vi "script-Matlab-proj.vi"(0 "Xr":i32[](array[numeric])=[230, 230, 230, 230, 230, 230, 230, 230, 230, 230, 230, 230, 230, 230, 230, 230, 230, 230, 230, 230, 230, 230, 230, 230, 230, 230, 230, 230, 230, 230, 230, 230, 230, 230, 230, 230, 230, 230, 230, 230, 230, 230, 230, 230, 230, 230, 230, 230, 230, 230, 230, 230, 230, 230, 230, 230, 230, 230, 230, 230, 230, 230, 230, 230, 230, 230, 230, 230, 230, 230, 225, 221, 213, 210, 206, 203, 195, 192, 189, 185, 179, 175, 172, 168, 162, 158, 155, 151, 145, 142, 139, 136, 129, 128, 131, 131, 136, 137, 139, 140, 144, 145, 147, 149, 151, 153, 155, 156, 159, 161, 163, 164, 167, 168, 170, 172, 175, 176, 178, 179, 182, 183, 184, 186, 189, 190, 191, 193, 195, 196, 198, 199, 201, 202, 203, 205, 207, 209, 209, 211, 213, 213], 1 "Xw":i32[](array[numeric])=[239, 239, 239, 239, 245, 265, 284, 302, 340, 359, 378, 397, 434, 453, 472, 491, 527, 545, 563, 580, 616, 635, 652, 670, 705, 723, 720, 705, 676, 663, 651, 641, 621, 612, 603, 595, 578, 569, 560, 552, 535, 526, 518, 509, 492, 484, 476, 467, 451, 442, 434, 426, 409, 401, 393, 385, 368, 360, 352, 344, 328, 320, 312, 304, 288, 280, 272, 264, 248, 241, 237, 234, 227, 223, 219, 215, 208, 204, 200, 197, 189, 186, 182, 178, 171, 167, 164, 160, 153, 149, 146, 143, 136, 132, 129, 128, 133, 135, 137, 138, 142, 144, 146, 147, 151, 152, 154, 156, 159, 161, 162, 164, 167, 168, 169, 171, 173, 175, 176, 178, 180, 181, 182, 184, 186, 187, 188, 190, 192, 193, 194, 195, 197, 198, 199, 200, 202, 203, 204, 205, 207, 208], 3 "filename":string="T5", 5 "Yr":i32[](array[numeric])=[319, 319, 319, 319, 319, 319, 319, 319, 319, 319, 319, 319, 319, 319, 319, 319, 319, 319, 319, 319, 319, 319, 319, 319, 319, 319, 319, 319, 319, 319, 319, 319, 319, 319, 319, 319, 319, 319, 319, 319, 319, 319, 319, 319, 319, 319, 319, 319, 319, 319, 319, 319, 319, 319, 319, 319, 319, 319, 319, 319, 319, 319, 319, 319, 319, 319, 319, 319, 319, 319, 315, 312, 306, 303, 301, 297, 291, 290, 287, 285, 280, 277, 274, 271, 267, 264, 261, 259, 255, 252, 249, 247, 242, 239, 239, 237, 233, 231, 229, 229, 225, 223, 222, 221, 217, 216, 214, 213, 210, 209, 207, 206, 203, 202, 200, 198, 195, 194, 193, 191, 189, 187, 187, 185, 183, 181, 180, 179, 176, 175, 174, 173, 171, 169, 168, 167, 165, 163, 163, 161, 159, 159], 9 "Xy":i32[](array[numeric])=[243, 243, 243, 243, 243, 243, 243, 243, 243, 243, 243, 243, 243, 243, 243, 243, 243, 243, 243, 243, 243, 243, 243, 243, 243, 243, 243, 243, 243, 243, 243, 243, 243, 243, 243, 243, 243, 243, 243, 243, 243, 243, 243, 243, 243, 243, 243, 243, 243, 243, 243, 243, 243, 243, 243, 243, 243, 243, 243, 243, 243, 243, 243, 243, 243, 243, 243, 243, 243, 243, 243, 243, 243, 243, 243, 243, 243, 243, 243, 243, 243, 243, 243, 243, 243, 243, 243, 243, 243, 243, 243, 243, 243, 243, 243, 243, 243, 243, 243, 243, 243, 243, 243, 243, 243, 243, 243, 243, 243, 243, 243, 243, 243, 243, 243, 243, 243, 243, 243, 243, 243, 243, 243, 243, 243, 243, 243, 243, 243, 243, 243, 243, 242, 242, 242, 242, 242, 242, 242, 242, 242, 242], 10 "error in":errorcluster, 11 "Yy":i32[](array[numeric])=[344, 344, 344, 344, 344, 344, 344, 344, 344, 344, 344, 344, 344, 344, 344, 344, 344, 344, 344, 344, 344, 344, 344, 344, 344, 344, 344, 344, 344, 344, 344, 344, 344, 344, 344, 344, 344, 344, 344, 344, 344, 344, 344, 344, 344, 344, 344, 344, 344, 344, 344, 344, 344, 344, 344, 344, 344, 344, 344, 344, 344, 344, 344, 344, 344, 344, 344, 344, 344, 344, 344, 344, 344, 344, 344, 344, 344, 344, 344, 344, 344, 344, 344, 344, 344, 344, 344, 344, 344, 344, 344, 344, 344, 344, 344, 344, 344, 344, 344, 344, 344, 344, 344, 344, 344, 344, 344, 344, 344, 344, 344, 344, 344, 344, 344, 344, 344, 344, 344, 344, 344, 344, 344, 344, 344, 344, 344, 344, 344, 344, 344, 344, 344, 344, 344, 344, 344, 344, 344, 344, 344, 344], 12 "Yw":i32[](array[numeric])=[368, 368, 368, 368, 369, 370, 372, 373, 377, 380, 382, 383, 387, 389, 391, 392, 391, 390, 389, 387, 386, 385, 384, 383, 381, 380, 382, 385, 390, 392, 391, 389, 386, 384, 383, 382, 379, 378, 376, 375, 373, 371, 370, 369, 367, 365, 364, 362, 360, 359, 357, 356, 354, 352, 351, 350, 347, 346, 345, 343, 341, 339, 338, 337, 335, 333, 332, 331, 328, 327, 329, 332, 336, 337, 339, 341, 344, 346, 348, 350, 353, 355, 356, 358, 361, 363, 365, 366, 369, 371, 373, 374, 378, 379, 381, 382, 383, 383, 384, 385, 386, 387, 388, 388, 390, 390, 391, 391, 392, 393, 393, 393, 393, 393, 393, 392, 391, 391, 391, 390, 390, 390, 389, 389, 388, 388, 388, 387, 387, 386, 386, 386, 386, 385, 385, 385, 384, 384, 384, 383, 383, 383], 13 "Line":string=".-", 14 "rgb1":string="68\t255\t18\n", 15 "rgb2":string="149\t0\t239\n") -> (4 "error out":errorcluster, 6 "matlab path":path=path "/Users/jammans/Documents/projet-prog/AnalyseT5.m")   [LabVIEW 2025]
panel:
  out "script matlab":string="% Auteurs: Rafaela Rebeiz, Jamil Mansour, Makram Fadel, Kevin Jandri\nclear\nclose all\nfilename = \"T5\";\nline = \".-\";\nrgb1 = [68\t255\t18\n];\nrgb2 = [149\t0\t239\n];\nXr=[230,230,230,230,230,230,230,230,230,230,230,230,230,230,230,230,230,230,230,230,230,230,230,230,230,230,230,230,230,230,230,230,230,230,230,230,230,230,230,230,230,230,230,230,230,230,230,230,230,230,230,230,230,230,230,230,230,230,230,230,230,230,230,230,230,230,230,230,230,230,225,221,213,210,206,203,195,192,189,185,179,175,172,168,162,158,155,151,145,142,139,136,129,128,131,131,136,137,139,140,144,145,147,149,151,153,155,156,159,161,163,164,167,168,170,172,175,176,178,179,182,183,184,186,189,190,191,193,195,196,198,199,201,202,203,205,207,209,209,211,213,213\n];\nYr=[319,319,319,319,319,319,319,319,319,319,319,319,319,319,319,319,319,319,319,319,319,319,319,319,319,319,319,319,319,319,319,319,319,319,319,319,319,319,319,319,319,319,319,319,319,319,319,319,319,319,319,319,319,319,319,319,319,319,319,319,319,319,319,319,319,319,319,319,319,319,315,312,306,303,301,297,291,290,287,285,280,277,274,271,267,264,261,259,255,252,249,247,242,239,239,237,233,231,229,229,225,223,222,221,217,216,214,213,210,209,207,206,203,202,200,198,195,194,193,191,189,187,187,185,183,181,180,179,176,175,174,173,171,169,168,167,165,163,163,161,159,159\n];\nXy=[243,243,243,243,243,243,243,243,243,243,243,243,243,243,243,243,243,243,243,243,243,243,243,243,243,243,243,243,243,243,243,243,243,243,243,243,243,243,243,243,243,243,243,243,243,243,243,243,243,243,243,243,243,243,243,243,243,243,243,243,243,243,243,243,243,243,243,243,243,243,243,243,243,243,243,243,243,243,243,243,243,243,243,243,243,243,243,243,243,243,243,243,243,243,243,243,243,243,243,243,243,243,243,243,243,243,243,243,243,243,243,243,243,243,243,243,243,243,243,243,243,243,243,243,243,243,243,243,243,243,243,243,242,242,242,242,242,242,242,242,242,242\n];\nYy=[344,344,344,344,344,344,344,344,344,344,344,344,344,344,344,344,344,344,344,344,344,344,344,344,344,344,344,344,344,344,344,344,344,344,344,344,344,344,344,344,344,344,344,344,344,344,344,344,344,344,344,344,344,344,344,344,344,344,344,344,344,344,344,344,344,344,344,344,344,344,344,344,344,344,344,344,344,344,344,344,344,344,344,344,344,344,344,344,344,344,344,344,344,344,344,344,344,344,344,344,344,344,344,344,344,344,344,344,344,344,344,344,344,344,344,344,344,344,344,344,344,344,344,344,344,344,344,344,344,344,344,344,344,344,344,344,344,344,344,344,344,344\n];\nXw=[239,239,239,239,245,265,284,302,340,359,378,397,434,453,472,491,527,545,563,580,616,635,652,670,705,723,720,705,676,663,651,641,621,612,603,595,578,569,560,552,535,526,518,509,492,484,476,467,451,442,434,426,409,401,393,385,368,360,352,344,328,320,312,304,288,280,272,264,248,241,237,234,227,223,219,215,208,204,200,197,189,186,182,178,171,167,164,160,153,149,146,143,136,132,129,128,133,135,137,138,142,144,146,147,151,152,154,156,159,161,162,164,167,168,169,171,173,175,176,178,180,181,182,184,186,187,188,190,192,193,194,195,197,198,199,200,202,203,204,205,207,208\n];\nYw=[368,368,368,368,369,370,372,373,377,380,382,383,387,389,391,392,391,390,389,387,386,385,384,383,381,380,382,385,390,392,391,389,386,384,383,382,379,378,376,375,373,371,370,369,367,365,364,362,360,359,357,356,354,352,351,350,347,346,345,343,341,339,338,337,335,333,332,331,328,327,329,332,336,337,339,341,344,346,348,350,353,355,356,358,361,363,365,366,369,371,373,374,378,379,381,382,383,383,384,385,386,387,388,388,390,390,391,391,392,393,393,393,393,393,393,392,391,391,391,390,390,390,389,389,388,388,388,387,387,386,386,386,386,385,385,385,384,384,384,383,383,383\n];\n\n\n% Main\n% Définir les constantes\n                                   \nSeqDateTime = datetime('now');       %faut changer ca ou le labview le change ?\nMoveDistPx = 9;                                     \nBallBorderDist = 9;\nCOLOR_R = 'r';\nCOLOR_Y = 'y';                             % pas trop necessaire, should we remove ?\nCOLOR_W = 'b';\n\n\n\nColor_touch_win = rgb1 / 255;\nColor_touch_loose = rgb2 / 255;\n\n% Nettoyer les données (NaN et outliers)\n[Xr, Yr] = InterpolateNan(Xr, Yr);\n[Xy, Yy] = InterpolateNan(Xy, Yy);\n[Xw, Yw] = InterpolateNan(Xw, Yw);\n\n[Xr, Yr] = RemoveOutlier(Xr, Yr);\n[Xy, Yy] = RemoveOutlier(Xy, Yy);\n[Xw, Yw] = RemoveOutlier(Xw, Yw);     %erreur a regler. On a white 41 px alors quil faut white 43 px    JUSTE CET ERREUR\n\ndisp(Xr);\ndisp(Yr);\n% Calculer le cadre\n[Xmin, Xmax, Ymin, Ymax] = GetFrame(Xr, Yr, Xy, Yy, Xw, Yw);\n\n% Calculer les longueurs de trajet\nPathR = GetBallPathLength(Xr, Yr);\nPathY = GetBallPathLength(Xy, Yy);\nPathW = GetBallPathLength(Xw, Yw);\n%disp(PathW);  test pour le nombre de white px !\n\n% Calculer l'ordre de mouvement\n[FirstBall, SecondBall, LastBall, NbBallsMoved] = GetBallMoveOrder(Xr, Yr, Xy, Yy, Xw, Yw, MoveDistPx); \n\n% get first move idx of each ball\n\nfirstmoveR = GetFirstMoveIdx(Xr, Yr, MoveDistPx);\nfirstmoveY = GetFirstMoveIdx(Xy, Yy, MoveDistPx);      % on peut supposer que par exemple la balle jaune touch la rouge a firstmoveR \nfirstmoveW = GetFirstMoveIdx(Xw, Yw, MoveDistPx);\n\ndisp('Indice first move = ');\ndisp(firstmoveR);\ndisp(firstmoveY);\ndisp(firstmoveW);\n\n\n% Trouver la première boule à bouger\n% Name1 is the first ball that moved\n\nif FirstBall == 1\n    Name1 = 'red';\n    Name1txt = 'r';\nelseif FirstBall == 2\n    Name1 = 'yellow';   \n    Name1txt = 'y';\nelseif FirstBall == 3\n    Name1 = 'white';\n    Name1txt = 'w';\nelse \n    Name1 = 'No ball moved'; % cas où aucune FirstBall = 0 \n    Name1txt ='N/A';\nend\n\n\n% Trouver les points de chocs\nif strcmp(Name1, 'red')  %check si Name1 = 'red'\n    touch = GetTouchIdx(Xr, Yr, Xmin, Xmax, Ymin, Ymax, BallBorderDist);\n    \nelseif strcmp(Name1, 'yellow')\n    touch = GetTouchIdx(Xy, Yy, Xmin, Xmax, Ymin, Ymax, BallBorderDist);      %est-ce ok de ne pas avoir le touchId de toutes les balles ? repponse : oui cest ok \n\nelseif strcmp(Name1, 'white')\n    touch = GetTouchIdx(Xw, Yw, Xmin, Xmax, Ymin, Ymax, BallBorderDist);\n\nelse\n    touch = [];   % si aucune balle ne bouge, pour pas avoir de error apres dans les plot\nend\n\n\n\n\ntouch_nb = length(touch);    \n\n% cherche si la balle a ganger ou perdu\n\n\nids = []; %stock nombre de toucher pour gagner\n\n\nif NbBallsMoved < 3    \n    WinLose = '---Lose---';\n    WinLosetxt = 'l';\nelse                       % on suppose donc ici que toute les boules bouge\n    if FirstBall == 1 \n        if SecondBall == 2\n            ids = find(touch > firstmoveY & touch < firstmoveW);\n        else \n            ids = find(touch > firstmoveW & touch < firstmoveY);\n        end\n    \n    elseif FirstBall == 2\n        if SecondBall == 1\n            ids = find(touch > firstmoveR & touch < firstmoveW);\n        else\n            ids = find(touch > firstmoveW & touch < firstmoveR);\n        end\n    \n    elseif FirstBall == 3 \n        if SecondBall == 1\n            ids = find(touch > firstmoveR & touch < firstmoveY);\n        else\n            ids = find(touch > firstmoveY & touch < firstmoveR);\n        end\n    end\n    \n    disp('Testing ids for win/lose = ');                 %% les indices que contient ids TRES TRES different des ids de touch, LOGIC\n    disp(ids);\n\n    number_touch = numel(ids);            %% ATTENTION, ici number_touch TRES TRES differnet de touch_nb, like number_touch always <= touch_nb\n    disp('number touch from ids = ');\n    disp(number_touch);\n    \n    if number_touch >= 3\n        WinLose = '---Win---';\n        WinLosetxt = 'w';\n    else\n        WinLose = '---Lose---';       % plus robuste, comme ca pas de risque de unrecognised variable\n        WinLosetxt = 'l';\n    end\nend\n\n\n    \n% SUPER DUPER IMPORTANT ∆∆∆∆∆∆∆∆∆∆∆∆               \n% ∆∆ ici on suppose que quand la boule touche une autre, elle bouge. Faut ask if assumption is correct or not et que si la balle touch other at indice, no way touch board at same id, so < and > enough\n                                                                         \n\n\n\n\n\n\n\n\n\n\n\n    \n\n%mais still besoin touchR, touchY, touchW au cas ou\n\n%touchR = GetTouchIdx(Xr, Yr, Xmin, Xmax, Ymin, Ymax, BallBorderDist);\n%touchY = GetTouchIdx(Xy, Yy, Xmin, Xmax, Ymin, Ymax, BallBorderDist);        % on peut enlever et juste dans le plot des chocs prend touch \n%touchW = GetTouchIdx(Xw, Yw, Xmin, Xmax, Ymin, Ymax, BallBorderDist);\n\n% 4. CRÉATION DU GRAPHIQUE\n%fprintf('Création du graphique...\\n');\n\nfig = figure('Name', 'Score Sheet', 'Color', 'k'); % Fenêtre avec fond noir\nhold on;\n\n% Tracer les trajectoires\nplot(Xr, 480 - Yr, line , 'Color', COLOR_R, 'LineWidth', 1);                          % How about the color ? Do we have to change here or the LabView will change it ?\nplot(Xy, 480 - Yy, line , 'Color', COLOR_Y, 'LineWidth', 1);                          % affichage faut changer de matlab ou bien le labview va les changer anyways ?\nplot(Xw, 480 - Yw, line , 'Color', COLOR_W, 'LineWidth', 1);\n\n% Tracer le cadre du billard\nW = Xmax - Xmin;\nH = Ymax - Ymin;\nrectangle('Position', [Xmin, 480 - Ymax, W, H], 'EdgeColor', 'b', 'LineWidth', 1);\n\n% Tracer les étoiles de position initiale\nplot(Xr(1), 480 - Yr(1), 'hexagram', 'MarkerSize', 20, 'MarkerEdgeColor', 'k');\nplot(Xy(1), 480 - Yy(1), 'hexagram', 'MarkerSize', 20, 'MarkerEdgeColor', 'k');     %LabVIEW choisi les shuriken\nplot(Xw(1), 480 - Yw(1), 'hexagram', 'MarkerSize', 20, 'MarkerEdgeColor', 'k');\n\n\n\n\n% Tracer les chocs (cercles)\n\nif strcmp(WinLose, '---Win---')\n\n    if strcmp(Name1, 'red')\n        plot(Xr(touch), 480 - Yr(touch), 'o', 'MarkerSize', 12, 'MarkerEdgeColor', Color_touch_win, 'LineWidth', 1);\n    \n    elseif strcmp(Name1, 'yellow')\n        plot(Xy(touch), 480 - Yy(touch), 'o', 'MarkerSize', 12, 'MarkerEdgeColor', Color_touch_win, 'LineWidth', 1);  \n    \n    elseif strcmp(Name1, 'white')\n        plot(Xw(touch), 480 - Yw(touch), 'o', 'MarkerSize', 12, 'MarkerEdgeColor', Color_touch_win, 'LineWidth', 1);\n    \n    end\n\nelse                                  % soit on gagne soit ou perd !         Mais elseif inside because we can have Name1 = 'No ball moved' !\n    \n    if strcmp(Name1, 'red')\n        plot(Xr(touch), 480 - Yr(touch), 'o', 'MarkerSize', 12, 'MarkerEdgeColor', Color_touch_loose, 'LineWidth', 1);\n    \n    elseif strcmp(Name1, 'yellow')\n        plot(Xy(touch), 480 - Yy(touch), 'o', 'MarkerSize', 12, 'MarkerEdgeColor', Color_touch_loose, 'LineWidth', 1);  \n    \n    elseif strcmp(Name1, 'white')\n        plot(Xw(touch), 480 - Yw(touch), 'o', 'MarkerSize', 12, 'MarkerEdgeColor', Color_touch_loose, 'LineWidth', 1);\n    \n    end\nend\n\n% Mise en forme du graphique\naxis equal; % Assure un ratio 1:1\naxis off;   % Cache les axes x/y\nset(gca, 'Color', 'w'); % Fond blanc\nset(gcf, 'Color', 'w');\nset(gcf, 'InvertHardcopy', 'off'); % Garde le fond noir lors de la sauvegarde\n\n% Ajouter le titre\ntitleStr = sprintf('Scores sheet - %s - %s', filename, SeqDateTime);\ntitle(titleStr, 'Color', 'k', 'FontSize', 14, 'FontWeight', 'bold');\n\n% Ajouter les annotations de texte (en bas)\nY_txt_line1 = Ymax + 10;\nY_txt_line2 = Ymax + 50;\nY_coord1 = 480 - Y_txt_line1;\nY_coord2 = 480 - Y_txt_line2;       %480 - : pour rammener le Y a notre repere 3ade\n\n\n\n\n\nwinnerStr = sprintf('Score sheet for \"%s\"\\n %s', Name1, WinLose);\ntext(Xmin, Y_coord1, winnerStr, 'Color', 'k', 'FontSize', 10, 'VerticalAlignment', 'top');\n\ndistStrR = sprintf('red_d:%dpx', round(PathR));\ntext(Xmin, Y_coord2, distStrR, 'Color', 'k', 'FontSize', 10, 'VerticalAlignment', 'top');             \n\ndistStrY = sprintf('yellow_d:%dpx', round(PathY));\ntext(Xmax / 2, Y_coord2, distStrY, 'Color', 'k', 'FontSize', 10, 'VerticalAlignment', 'top');\n\ndistStrW = sprintf('white_d:%dpx', round(PathW));\ntext(Xmax, Y_coord2, distStrW, 'Color', 'k', 'FontSize', 10, 'VerticalAlignment', 'top', 'HorizontalAlignment', 'right');\n\nsummaryStr = sprintf('%d ball(s) moved\\n%d band(s) touched', NbBallsMoved, touch_nb);\ntext(Xmax, Y_coord1, summaryStr, 'Color', 'k', 'FontSize', 10, 'VerticalAlignment', 'top', 'HorizontalAlignment', 'right');\n\nhold off;\n\n% 5. SAUVEGARDE DES RÉSULTATS\n%fprintf('Sauvegarde des résultats...\\n');\n\n% Sauvegarder l'image en PDF\npdfFileName = sprintf('ScoreSheet%s.pdf', filename);\nprint(fig, pdfFileName, '-dpdf', '-fillpage');\nfprintf('Graphique sauvegardé en : %s\\n', pdfFileName);\n\n% Sauvegarder le résumé en TXT\ntxtFileName = sprintf('Summary%s.txt', filename);\nfid = fopen(txtFileName, 'w');\nif fid == -1\n    error('Impossible de créer le fichier TXT.');\nend\n\n% fprintf(fid, '--- Summary for %s - %s ---\\n\\n', filename, SeqDateTime);\n% fprintf(fid, 'Winner: %s (Balle %d)\\n', Name1, FirstBall);\n% fprintf(fid, 'Balls Moved: %d\\n', NbBallsMoved);\n% fprintf(fid, 'Bands Touched: %d\\n\\n', touch_nb);\n% fprintf(fid, '--- Path Lengths ---\\n');                                    \n% fprintf(fid, '  Red:    %d px\\n', round(PathR));\n% fprintf(fid, '  Yellow: %d px\\n', round(PathY));\n% fprintf(fid, '  White:  %d px\\n\\n', round(PathW));\n% fprintf(fid, '--- File Generated ---\\n');\n% fprintf(fid, 'ScoreSheet PDF: %s\\n', pdfFileName);\n\nfprintf(fid, 'f:%s; ',Name1txt);\nfprintf(fid, 's:%s; ',WinLosetxt);\nfprintf(fid, 'n:%d; ',NbBallsMoved);\nfprintf(fid, 'b:%d; ',touch_nb);\nfprintf(fid, 'rb:%d; ',round(PathR));\nfprintf(fid, 'yb:%d; ',round(PathY));\nfprintf(fid, 'wb:%d; ',round(PathW));\n\n\n\nfclose(fid);\nfprintf('Résumé sauvegardé en : %s\\n', txtFileName);\n\n%fprintf('Analyse terminée.\\n');\n\n\n% ########################################################################\n%\n%  DEFINITION DES FONCTIONS LOCALES\n%\n% ########################################################################\n\n% ajouter arbitrairement un\t'0'\tou\tautre\tvaleur\tpertinente dans le cas\n% ou on a NaN au debut et/ou a la fin\n\n% EXO 4\nfunction [X, Y] = InterpolateNan(X,Y)\n    added_start = false;\n    added_end = false;\n    if isnan(X(1))\n        X = [0 , X];\n        Y = [0 , Y];\n        added_start = true;\n    end\n    \n    if isnan(X(end))\n        X(end + 1) = 0;\n        Y(end + 1) = 0;\n        added_end = true; \n    end\n    \n    idx_connus_X = find(~isnan(X));\n    \n    valeurs_connues_X = X(idx_connus_X);\n    \n    idx_tous_X = 1:length(X);\n    X = interp1(idx_connus_X, valeurs_connues_X, idx_tous_X, 'next');\n    idx_connus_Y = find(~isnan(Y));\n    \n    valeurs_connues_Y = Y(idx_connus_Y);\n    \n    idx_tous_Y = 1:length(Y);\n    Y = interp1(idx_connus_Y, valeurs_connues_Y, idx_tous_Y, 'next');\n    if added_start\n        X = X(2:end);\n        Y = Y(2:end);\n    end\n    if added_end\n        X = X(1:end-1);\n        Y = Y(1:end-1);\n    end\n    \nend\n%%% QUESTION SUPER IMPORTANTE AUX ASSISTANTS: est ce que cest possible\n%%% davoir un outlier au premier element?   ATTENTION BOUCLE FOR\n\n%%%%% Voir en bas pourquoi j'ai comment-out cette partie\n\n% function [X,Y] = RemoveOutlier(X, Y)\n%     outlierX = isoutlier(X, 'movmedian', 10);\n% \n%     outlierY = isoutlier(Y, 'movmedian', 10);\n%     idx_out_X = find(outlierX);\n%     idx_out_Y = find(outlierY);\n% \n%     % Remplacer pour X (en gérant le cas de l'index 1)\n%     for i = 1:length(idx_out_X)\n%         idx = idx_out_X(i); % L'index de l'outlier actuel\n%         if idx > 1\n%             X(idx) = X(idx - 1); % Cas normal: on prend le précédent\n%         else\n%             % Cas spécial: l'outlier EST à l'index 1\n%             X(idx) = X(idx + 1); % On prend le suivant\n%         end\n%     end\n% \n%     % Remplacer pour Y (en gérant le cas de l'index 1)\n%     for i = 1:length(idx_out_Y)\n%         idx = idx_out_Y(i);\n%         if idx > 1\n%             Y(idx) = Y(idx - 1);\n%         else\n%             Y(idx) = Y(idx + 1);\n%         end\n%     end\n% end\n\n\n%%%% Mak ici RemoveOutlier() mais sans BOUCLE FOR ni 1st as Outlier\n%%%% Akid faut ask assistant bass si on compte 1st as Outlier, on a pas\n%%%% le bon schema a la fin. On a un truc faux. J'ai test et au lieu de 700\n%%%% et 300 pour premier coord, ca donnai celle dapres, et on perdait le\n%%%% first shoot en sa totalite.\n\n\nfunction[X,Y] = RemoveOutlier(X, Y)\n\noutlierX = isoutlier(X, 'movmedian', 10);\noutlierY = isoutlier(Y, 'movmedian', 10);\n\noutlierX([1 end]) = false;\noutlierY([1 end]) = false;\n\nidx_out_X = find(outlierX);    %done les index ou ya les outliers dans X\nX(idx_out_X) = X(idx_out_X - 1);  %remplace valeur outlier par precedente valeur ie (-1)\n\nidx_out_Y = find(outlierY);       %pas de risque outofrange  car 1 et end = false (hypo,ask assistant)\nY(idx_out_Y) = Y(idx_out_Y - 1);    % pas de probleme de faire -1 car ya pas de groupe de outlier !\n\n% pas besoin de call plusieurs fois avec for, idx_out_X donne tous les\n% index a changer direct. Magie du Maklab !\nend\n\n%%%%%% Exo 1: Plot de la trajectoire de chaque balle %%%%%%%\n% (Cette partie est maintenant gérée par le script principal ci-dessus)\n% plot(Xr, 480 -Yr , 'r', 'LineWidth', 2);\n% ...\n% rectangle('Position', [Xmin, 480-Ymax, W, H], ...\n%           'EdgeColor','w', 'LineWidth',1.5);\n\n%%%%%%% Exo 2 question 1 %%%%%%%%%\n% Rq: demander si cest ok de call la fonction avant que l'on ne la definit\nfunction [Xmin, Xmax, Ymin, Ymax] = GetFrame(Xr, Yr, Xy, Yy, Xw, Yw)\n    all_X = [Xr, Xy, Xw];\n    all_Y = [Yr, Yy, Yw];\n    \n    Xmin = min(all_X);\n    Xmax = max(all_X); %calcul min et max global\n    Ymin = min(all_Y);\n    Ymax = max(all_Y);\nend\n%%%%%% Exo 2 question 2 %%%%%%%%\nfunction PathLength = GetBallPathLength(X,Y)\n    \n    norme = sqrt(diff(X).^2 + diff(Y).^2);\n    PathLength = sum(norme); \n\nend\n% (Appels maintenant gérés par le script principal)\n% GetBallPathLength(Xr,Yr);\n% GetBallPathLength(Xy,Yy);    % j'ai tester, les valeurs sont OK          \n% GetBallPathLength(Xw,Yw);\n\n%%%%%%%% Exo 2 question 3 %%%%%%%\n% function FirstMoveIdx = GetFirstMoveIdx(X,Y, MoveDistPx)\n %   deltaX = X - X(1);\n  %  deltaY = Y - Y(1);              %ATTENTION :FAUX(voir en bas pour explication)\n   % distances = sqrt(diff(deltaX).^2 + diff(deltaY).^2);\n    %FirstMoveIdx = find(distances > MoveDistPx, 1 , 'first');\n%end\n % Mak dans lexo 3 il demande de changer GetFirstMove. C'est pour ca que ca a\n% changer compare a avant\n\nfunction [FirstMoveIdx, MoveDist] = GetFirstMoveIdx(X, Y, MoveDistPx)\n   \n\n    MoveDist = sqrt(diff(X.^2) + diff(Y.^2));    % This shouldn't work , because as the prof said, we take 1st segment and 1st segment is sometimes equal 0. like in this exemple. It should be MoveDist = distance\n                                                 % Because we should look\n                                                 % at first distance after\n                                                 % collision, not overall\n    X = X - X(1);                        % change de referentiel                                               ∆∆∆∆∆∆∆∆∆∆∆∆∆∆∆∆∆∆∆∆∆∆∆∆∆∆∆∆∆∆∆∆∆∆∆∆∆∆∆∆∆∆∆∆∆∆∆∆∆∆∆∆∆∆∆∆∆∆∆∆∆∆∆∆∆∆∆∆∆∆∆∆∆∆∆∆∆∆\n    Y = Y - Y(1);\n    distance = sqrt(X.^2 + Y.^2);                   % pas besoin de faire diff car p.i. est (0,0)   %%CHANGER MoveDist avec distance\n                                                    % apres avoir changer referentiel\n    FirstMoveIdx = find(distance > MoveDistPx, 1 , 'first');\n    \n    % MoveDist = sqrt(diff(X.^2) + diff(Y.^2)); % ici, cest dist parcourut segment par segment      QUESTION : MoveDist doit rester comme ca, avec le X = X - X(1) ? Ou faut changer et remettre X = X + X(1) ?\n    \n    %MoveDist = distance;\n    \n    % if emtpy (...) pas necessaire, car find va auto donne [] vide si pas\n    % trouve\nend\n% EXPLICATION\n% GetFirstMoveIdx renvoie la position dans le array (index i) tel\n% que la ball a bouger pour la premiere fois (d'ou FirstMoveIdx)\n% Ne pas oublier que sur Maklab, les arrays comment par 1 et non pas 0 !\n% La fonction renvoie 4 pour rouge, 2 pour yellow, et 102 pour blanche, ce\n% qui est parfaitement logique. J'ai aussi check avec des made up valeurs,\n% c'est all good. La fonction qu'on avait fait avait donne de fausses valeurs\n% d'indice, parce qu'on faisait diff() dans le calcul de distance.\n% Ce n'est enfaite pas necessaire puisque on a deja changer le referentiel\n% pour faire en sorte que la postion initial est (0,0). Et comme x-0 = x, ya\n% pas besoin de faire diff(), sinon cela fausse les resultat.\n% La version correct est celle ci, celle SANS les diff(). \n\n% (Appels maintenant gérés par le script principal)\n% firstMoveIdxR = GetFirstMoveIdx(Xr, Yr, 9);\n% firstMoveIdxY = GetFirstMoveIdx(Xy, Yy, 9);\n% firstMoveIdxW = GetFirstMoveIdx(Xw, Yw, 9);\n% disp(firstMoveIdxR);\n% disp(firstMoveIdxY);     % juste des petits test\n%disp(firstMoveIdxW);\n\n%%%%%%%% Exo 3 question 1 %%%%%%%\nfunction [IdxTouch] = GetTouchIdx(X, Y, Xmin, Xmax, Ymin, Ymax, BallBorderDist)\n    idxLeft = find(X - Xmin <= BallBorderDist);\n    idxRight = find(Xmax - X <= BallBorderDist);     % Attention:faut ni mettre 1, ni 'first'\n    idxTop = find(Y - Ymin <= BallBorderDist);       % Pas besoin de abs (ask au cas ou) \n    idxBottom = find(Ymax - Y <= BallBorderDist);    \n    % dans cette fonction, il ya 2 choses a checker. Si deux bords sont hit\n    % successivement et Si deux boules satisfont la condition du find.\n    % Ce sont deux cas differents, quon ne peut pas check d'un seul coup.\n    % On commence d'abord par check chaque bord seule si on a des index\n    % successifs. Sinon, si je check apres tout avoir mit ensemble, je risk\n    % de perdre des rebonds sur des bords successif, qui se feront passer\n    % pour des doublons qui satisfait la condition <= BallBorder Dist\n    % Voir SUPER IMPORTANT en bas pour remarque\n    % ask about\n                                                        % abs() ?\n                                                         % SUPER IMPORTANT\n \n    if ~isempty(idxLeft)                                   % Truc du 1er idx\n        idxLeft = idxLeft([true, diff(idxLeft) > 1]);      % true, cest pour ajouter\n    end\n    if ~isempty(idxRight) \n        idxRight = idxRight([true, diff(idxRight) > 1]);       % true au vecteur logique                                             \n    end\n    if ~isempty(idxTop) \n        idxTop = idxTop([true, diff(idxTop) > 1]);             % comme ca on ne prend que\n    end\n    if ~isempty(idxBottom) \n        idxBottom = idxBottom([true, diff(idxBottom) > 1]);    % 1er indice SUPER IMPORTANT\n    end\n    %%% Rq: demander aux assistant si les idx correspondent bien aux index de la listr Xr ou Yr     \n    %%%%% et si l'order des index est important ou pas(ex: 23 79 10 67 28)       \n    [IdxTouch] = [idxLeft idxRight idxTop idxBottom];  % on fusionne le tout\n    [IdxTouch] = unique(IdxTouch);  % enleve les doublons.'Stable' doesn't change order            faut demander si on garde stable ou si on tri en ordre croissant \n   \n    IdxTouch(IdxTouch == 1) = [];             % enelve index = 1\n  \nend\n%%% SUPER IMPORTANT: question assistant : Par prendre la premiere, on veut\n%%% dire prendre la premiere de gauche a droite ou de droite a gauche ?\n%%% Ou bien adapte a chaque cas ?\n%%%% IMPORTANT !!!!!\n%%% ie: le 1er qui verifie la condition ou le premier qui touche le bord???\n%%%% IMPORTANT !!!!!\n%%% Car prendre la premiere a droite != premiere a gauche   !!!!!!\n%%% Est-ce que Valeur Absolue resout le problem ?????\n\n% (Appels maintenant gérés par le script principal)\n% disp(GetTouchIdx(Xr, Yr, Xmin, Xmax, Ymin, Ymax, 9));\n% disp(GetTouchIdx(Xy, Yy, Xmin, Xmax, Ymin, Ymax, 9));\n% disp(GetTouchIdx(Xw, Yw, Xmin, Xmax, Ymin, Ymax, 9)); %renvoie rien car on a []\n                                                      %car balle blanche\n                                                      %touche pas bord ici\n                                                     \nfunction [FirstBall,SecondBall,LastBall, NbBallsMoved] = GetBallMoveOrder(Xr, Yr, Xy, Yy, Xw, Yw, MoveDistPx)\n    def_idx = [1 2 3]; % red = 1, yellow = 2 , white = 3\n    [idxR,segsR] = GetFirstMoveIdx(Xr, Yr, MoveDistPx);\n    [idxY,segsY] = GetFirstMoveIdx(Xy, Yy, MoveDistPx);\n            \n    [idxW,segsW] = GetFirstMoveIdx(Xw, Yw, MoveDistPx);\n    \n    len = length(Xr); % Longueur de référence\n    if isempty(idxR), idxR = len + 1; end\n    if isempty(idxY), idxY = len + 1; end   % on fait ca puisque si cest vide,[] abime tout\n    if isempty(idxW), idxW = len + 1; end\n    \n    d1R = 0;\n    d1Y = 0;  % variable pour stocker distance initial parcourue\n    d1W = 0;\n    fprintf('idxR=%s, idxY=%s, idxW=%s\\n', mat2str(idxR), mat2str(idxY), mat2str(idxW));\n    if ~isempty(segsR), d1R = segsR(1); end      %%% ici est-ce que idxR idxY idxW or 1 1 1 ???? ∆∆∆∆     %le prof a dit 1 1 1, (1er segment). Maybe add a condition if all = 0 ?\n    if ~isempty(segsY), d1Y = segsY(1); end  % si non vide, donne aux variables d1, sinon reste 0\n    if ~isempty(segsW), d1W = segsW(1); end\n    fprintf('d1R=%.3f, d1Y=%.3f, d1W=%.3f\\n', d1R, d1Y, d1W);\n    \n    store_idx = [idxR idxY idxW];                                                                                   %Documentation hyper important ici ∆∆∆∆∆\n    store_d1 = [d1R d1Y d1W];                 %∆∆∆ le 1 et le 2 sont les COLONNES UTILISE POUR TRIER LA MATRICE, le - cest pour dire dans l'ordre decroissant car on veut les plus grandes distances au debut ∆∆∆\n                                                      %bien sur que la ligne suit le trie de la colonne. SO BASICALLY ON UTILISE LES ELEMENTS DE LA COLONNE # POUR BOUGER LES LIGNES DE LA MATRICE                                                                  \n    M = [store_idx(:) store_d1(:) def_idx(:)];   %% trie d'abord selon la colonne 1 dans l'ordre croissant, boule qui bouge en premier a le plus petit indice et donc est au debut de la colonne 1     \n    M = sortrows(M, [1 -2]);                     %% Ensuite si deux lignes on la meme valeur dans la colonne 1 ie: on a le meme indice, alors on trie encore la matrice suivant la 2eme colonne\n                                                                         % ET LES SEULES LIGNES QUI BOUGENT SONT CELLES OU DANS LA COLONNE 1 YA UNE EGALITE !\n    moved_ids = M(M(:,1) <= len, 3).'; % Filtre en utilisant 'len' et les valeur de la premiere colonne \n    NbBallsMoved = numel(moved_ids);\n    % numel cest number of elements \n    disp(100001);\n    disp(moved_ids);\n    FirstBall = 0; SecondBall = 0; LastBall = 0;\n    if NbBallsMoved >= 1, FirstBall = moved_ids(1); end     \n    if NbBallsMoved >= 2, SecondBall = moved_ids(2); end\n    if NbBallsMoved >= 3, LastBall = moved_ids(3); end\n   \nend\n\n%Pour Documentation:\n%POUR SORTROWS\n% On trie d'abord toutes les lignes selon les valeurs de la colonne 1.\n% Si egalite, on trie alors les lignes ou ya des valeurs egales \n% (et seulement ces lignes) selon les valeurs de la colonne 2, \n% en ordre decroissant.\n%\n%\n%POUR moved_ids\n%colonne 1 deja trier, creer un vecteur logique \n%puis on garde les cases de colonne 3 ou c'est TRUE\n%[true, false, true] on garde [ case 1, case 3]\n%\n%\n% Version 1 Decembre 2:00 PM \n%\n% \n\n\n\n"
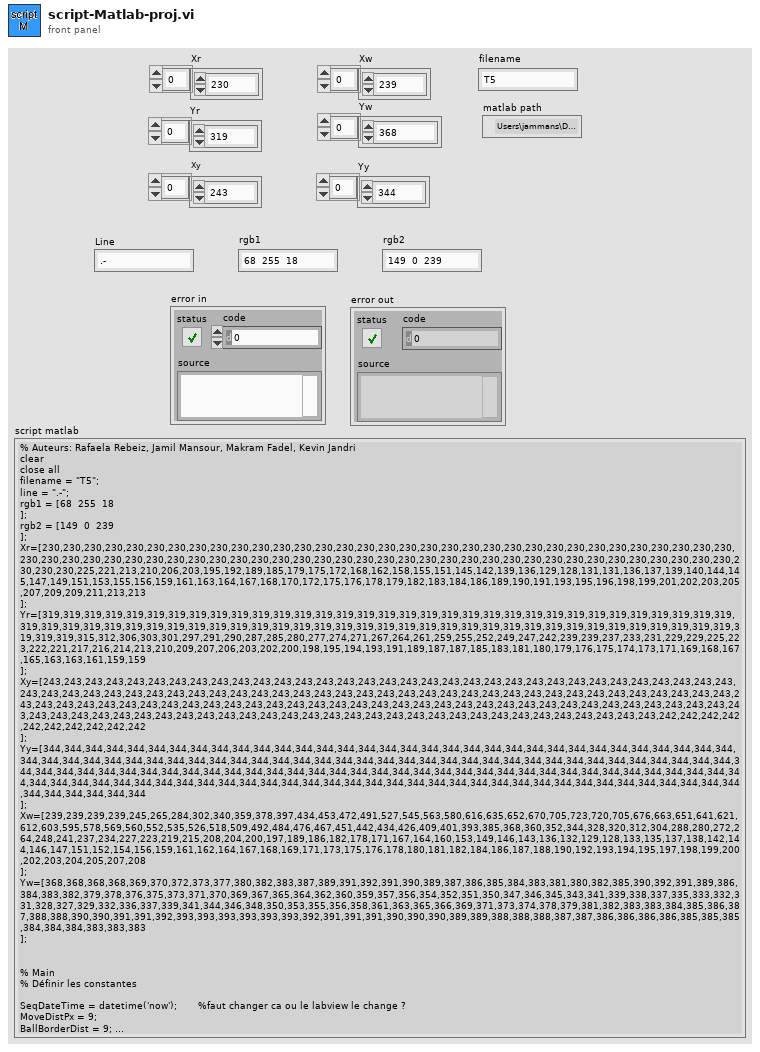
[diagram p1: front panel]
types:
  T1 = enum16{"open", "replace", "create", "open or create", "replace or create", "replace or create with confirmation"}
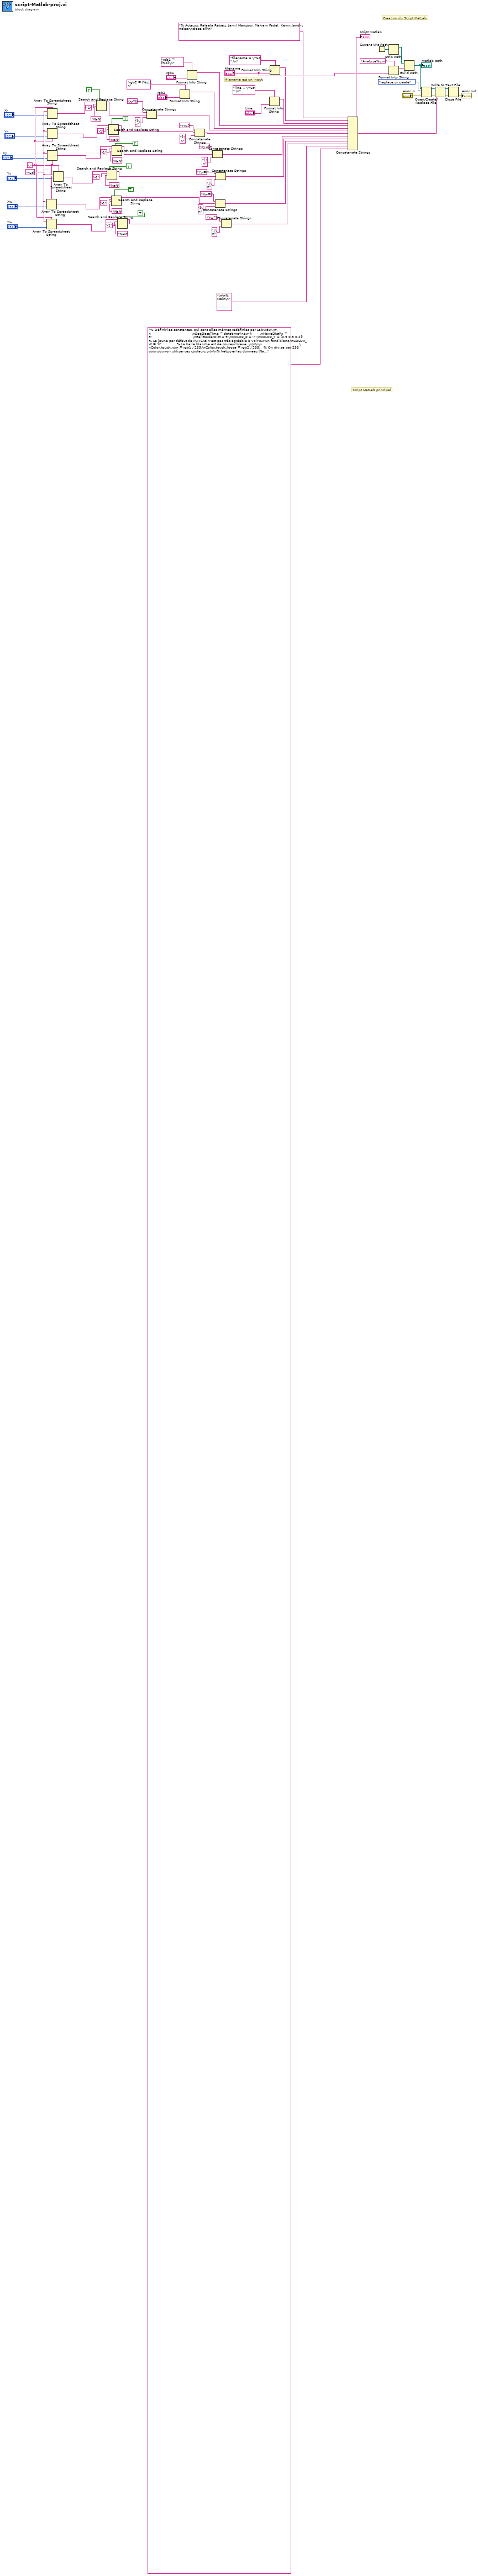
[diagram p0: block diagram]
diagram:
  w81 = "," ("delimiter (Tab)")
  w82 = "%d" ("format string")
  # "Script MatLab principal"
  # "Creation du Script MatLab"
  # "filename est un input"
  n1 = Array To Spreadsheet String(delimiter (Tab)=w81, array="Xw", 3:w82) -> (spreadsheet string=w22:string)
  n2 = Array To Spreadsheet String(delimiter (Tab)=w81, array="Yw", 3:w82) -> (spreadsheet string=w18:string)
  n3 = Array To Spreadsheet String(delimiter (Tab)=w81, array="Xr", 3:w82) -> (spreadsheet string=w40:string)
  n4 = Array To Spreadsheet String(delimiter (Tab)=w81, array="Yr", 3:w82) -> (spreadsheet string=w34:string)
  n5 = Array To Spreadsheet String(delimiter (Tab)=w81, array="Xy", 3:w82) -> (spreadsheet string=w30:string)
  n6 = Array To Spreadsheet String(delimiter (Tab)=w81, array="Yy", 3:w82) -> (spreadsheet string=w26:string)
  n7 = Search and Replace String(replace all?=TRUE ("replace all? (F)"), input string=w40, search string="-1", replace string="NaN" ("replace string (\"\")")) -> (result string=w37:string)  [unwired: 4 in, 3 out]
  n8 = Search and Replace String(replace all?=TRUE ("replace all? (F)"), input string=w26, search string="-1", replace string="NaN" ("replace string (\"\")")) -> (result string=w25:string)  [unwired: 4 in, 3 out]
  n9 = Search and Replace String(replace all?=TRUE ("replace all? (F)"), input string=w34, search string="-1", replace string="NaN" ("replace string (\"\")")) -> (result string=w33:string)  [unwired: 4 in, 3 out]
  n10 = Search and Replace String(replace all?=TRUE ("replace all? (F)"), input string=w22, search string="-1", replace string="NaN" ("replace string (\"\")")) -> (result string=w21:string)  [unwired: 4 in, 3 out]
  n11 = Search and Replace String(replace all?=TRUE ("replace all? (F)"), input string=w30, search string="-1", replace string="NaN" ("replace string (\"\")")) -> (result string=w29:string)  [unwired: 4 in, 3 out]
  n12 = Search and Replace String(replace all?=TRUE ("replace all? (F)"), input string=w18, search string="-1", replace string="NaN" ("replace string (\"\")")) -> (result string=w17:string)  [unwired: 4 in, 3 out]
  n13 = Concatenate Strings("Xr=[" ("string"), w37, "];\n" ("string")) -> (w76:string)
  n14 = Format Into String(format string="rgb2 = [%s];\n", "rgb2") -> (resulting string=w2:string)  [unwired: 2 in, 1 out]
  n15 = Format Into String(format string="rgb1 = [%s];\n", "rgb1") -> (resulting string=w3:string)  [unwired: 2 in, 1 out]
  n16 = Concatenate Strings("Yr=[" ("string"), w33, "];\n" ("string")) -> (w73:string)
  n17 = Concatenate Strings("Xy=[" ("string"), w29, "];\n" ("string")) -> (w70:string)
  n18 = Concatenate Strings("Xw=[" ("string"), w21, "];\n" ("string")) -> (w64:string)
  n19 = Concatenate Strings("Yy=[" ("string"), w25, "];\n" ("string")) -> (w67:string)
  n20 = Concatenate Strings("Yw=[" ("string"), w17, "];\n" ("string")) -> (w61:string)
  n21 = Format Into String(format string="line = \"%s\";\n" ("input 6"), "Line") -> (resulting string=w8:string)  [unwired: 2 in, 1 out]
  n22 = Format Into String(format string="filename = \"%s\";\n", "filename") -> (resulting string=w9:string)  [unwired: 2 in, 1 out]
  n23 = Concatenate Strings("% Auteurs: Rafaela Rebeiz, Jamil Mansour, Makram Fadel, Kevin Jandri\nclear\nclose all\n", w9, w8, w3, w2, w76, w73, w70, w67, w64, w61, "\n\n% Main\n", "% Définir les constantes, qui sont elles-mêmes redéfinies par LabVIEW.\n\n                                     \nSeqDateTime = datetime('now');       \nMoveDistPx = 9;                                     \nBallBorderDist = 9;\nCOLOR_R = 'r';\nCOLOR_Y = [0.9 0.8 0.2];   % Le jaune par défaut de MATLAB n'est pas très agréable à voir sur un fond blanc.\nCOLOR_W = 'b';             % La balle blanche est de couleur bleue. \n\n\n\n                                  \nColor_touch_win = rgb1 / 255;\nColor_touch_loose = rgb2 / 255;   % On divise par 255 pour pouvoir utiliser ces couleurs.\n\n\n% Nettoyer les données (NaN et Outliers)\n\n[Xr, Yr] = InterpolateNan(Xr, Yr);\n[Xy, Yy] = InterpolateNan(Xy, Yy);\n[Xw, Yw] = InterpolateNan(Xw, Yw);\n\n[Xr, Yr] = RemoveOutlier(Xr, Yr);\n[Xy, Yy] = RemoveOutlier(Xy, Yy);\n[Xw, Yw] = RemoveOutlier(Xw, Yw);     \n\n\n% Calculer le cadre \n\n[Xmin, Xmax, Ymin, Ymax] = GetFrame(Xr, Yr, Xy, Yy, Xw, Yw);\n\n% Calculer les longueurs de trajet\n\nPathR = GetBallPathLength(Xr, Yr);\nPathY = GetBallPathLength(Xy, Yy);\nPathW = GetBallPathLength(Xw, Yw);\n\n\n\n% Calculer l'ordre de mouvement\n\n[FirstBall, SecondBall, LastBall, NbBallsMoved] = GetBallMoveOrder(Xr, Yr, Xy, Yy, Xw, Yw, MoveDistPx); \n\ndisp(' ');\ndisp('Ordre de mouvement : ')\ndisp(' ');\ndisp('FirstBall = ');\ndisp(FirstBall);\n\ndisp('SecondBall = ');\ndisp(SecondBall);                % Si une balle ne bouge pas, valeur = 0 \n                                 % Convention :   \ndisp('LastBall = ');             % Red = 1 Yellow = 2 White = 3\ndisp(LastBall);\n\ndisp('NbBallsMoved = ');\ndisp(NbBallsMoved);\n\n\n\n% Get first move idx of each ball\n\nfirstmoveR = GetFirstMoveIdx(Xr, Yr, MoveDistPx);\nfirstmoveY = GetFirstMoveIdx(Xy, Yy, MoveDistPx);      % Note: On suppose que par exemple la balle jaune (FirstBall) touche la rouge a firstmoveR \nfirstmoveW = GetFirstMoveIdx(Xw, Yw, MoveDistPx);            % et la blanche à firstmoveW, donc une 2nd ball et 3rd ball ne bouge que lorsqu'elles\n                                                             % sont touchées par 1st Ball\n                                                             \n                                                             \ndisp('Indices first move : ');\ndisp(' ');\ndisp('Red = ');\ndisp(firstmoveR);\ndisp('Yellow = ');                 % Si une balle ne bouge pas, valeur = []\ndisp(firstmoveY);\ndisp('White = ');\ndisp(firstmoveW);\n\n\n% Trouver la première boule à bouger\n% Name1 is the first ball that moved\n\nif FirstBall == 1\n    Name1 = 'red';\n    Name1txt = 'r';\nelseif FirstBall == 2\n    Name1 = 'yellow';   \n    Name1txt = 'y';\nelseif FirstBall == 3\n    Name1 = 'white';\n    Name1txt = 'w';\nelse \n    Name1 = 'No ball moved'; % cas où aucune balle ne bouge\n    Name1txt ='N/A';\nend\n\n\n% Trouver TOUS les points de chocs \nif strcmp(Name1, 'red')  % strcmp() check si Name1 = 'red'\n    touch = GetTouchIdx(Xr, Yr, Xmin, Xmax, Ymin, Ymax, BallBorderDist);      % GetTouchIdx prend TOUS les rebonds.\n    \nelseif strcmp(Name1, 'yellow')\n    touch = GetTouchIdx(Xy, Yy, Xmin, Xmax, Ymin, Ymax, BallBorderDist);       \n                                                                             \nelseif strcmp(Name1, 'white')\n    touch = GetTouchIdx(Xw, Yw, Xmin, Xmax, Ymin, Ymax, BallBorderDist);\n\nelse\n    touch = [];   % si aucune balle ne bouge, pour pas avoir de errors après dans les plots\nend\n\n\ndisp('Touch idexes with no filtering (TOTAL TOUCHES) = ');\ndisp(touch);\n    \n\n% Test si la balle Win or Lose\n\n\n\nif NbBallsMoved < 3    \n    WinLose = '---Lose---';       % Notre convention : Si pas toutes les balles bouges (donc Lose), on va juste prendre TOUS LES REBONDS de la boule, on ne filtre pas touch.\n    WinLosetxt = 'l';\n\n    touch_nb = numel(touch);\n\n    disp('Number of Touches TOTAL (cas où NbBallsMoved < 3, no filtering)  = ');\n    disp(touch_nb);\n\n    % disp (touch) pas nécessaire car déjà fait en haut, et touch reste le\n    % même\n\nelse                       % On suppose donc ici que toutes les boules bougent, donc on filtre touch : on ne garde que les indices entre les indices de SecondBall et LastBall\n    if FirstBall == 1 \n        if SecondBall == 2\n            touch = touch(touch >= firstmoveY & touch <= firstmoveW);\n        else \n            touch = touch(touch >= firstmoveW & touch <= firstmoveY);         \n        end\n    \n    elseif FirstBall == 2\n        if SecondBall == 1\n            touch = touch(touch >= firstmoveR & touch <= firstmoveW);         \n        else\n            touch = touch(touch >= firstmoveW & touch <= firstmoveR);\n        end\n    \n    elseif FirstBall == 3 \n        if SecondBall == 1\n            touch = touch(touch >= firstmoveR & touch <= firstmoveY);\n        else\n            touch = touch(touch >= firstmoveY & touch <= firstmoveR);\n        end\n    end\n    \n    disp('Touch filtered = ');                 % Ici on n'a pas touch TOTAL, mais touch entre 2ème et 3ème boule\n    disp(touch);\n\n    touch_nb = numel(touch);            \n    \n    disp('Number of Touch filtered = ');       % Nombre de touch entre 2ème et 3ème boule\n    disp(touch_nb);\n    \n    if touch_nb >= 3\n        WinLose = '---Win---';\n        WinLosetxt = 'w';\n    else\n        WinLose = '---Lose---';               % plus robuste, pas de risque de unrecognised variable\n        WinLosetxt = 'l';\n    end\nend\n\n\n    \n\n% Note: On suppose que la SecondBall et LastBall bouge seulement lorsque\n% la FirstBall les touche.\n\n% Voir aussi documentation pour les choix de touch et touch_nb selon les\n% cas\n\n\n    \n\n% 4. CRÉATION DU GRAPHIQUE\n\nfig = figure('Name', 'ScoreSheet', 'Color', 'w');    % pour voir résultat directement sur MatLab\nhold on;\n\n% Tracer les trajectoires\nplot(Xr, 480 - Yr, line , 'Color', COLOR_R, 'LineWidth', 1);                          \nplot(Xy, 480 - Yy, line , 'Color', COLOR_Y, 'LineWidth', 1);                          \nplot(Xw, 480 - Yw, line , 'Color', COLOR_W, 'LineWidth', 1);\n\n% Tracer le cadre du billard\nW = Xmax - Xmin;\nH = Ymax - Ymin;\nrectangle('Position', [Xmin, 480 - Ymax, W, H], 'EdgeColor', 'b', 'LineWidth', 1);\n\n% Tracer les étoiles de position initiale\nplot(Xr(1), 480 - Yr(1), 'hexagram', 'MarkerSize', 15, 'MarkerEdgeColor', 'k');\nplot(Xy(1), 480 - Yy(1), 'hexagram', 'MarkerSize', 15, 'MarkerEdgeColor', 'k');     \nplot(Xw(1), 480 - Yw(1), 'hexagram', 'MarkerSize', 15, 'MarkerEdgeColor', 'k');\n\n\n\n\n% Tracer les chocs (cercles)\n\nif strcmp(WinLose, '---Win---')\n\n    if strcmp(Name1, 'red')\n        plot(Xr(touch), 480 - Yr(touch), 'o', 'MarkerSize', 15, 'MarkerEdgeColor', Color_touch_win, 'LineWidth', 1);\n    \n    elseif strcmp(Name1, 'yellow')\n        plot(Xy(touch), 480 - Yy(touch), 'o', 'MarkerSize', 15, 'MarkerEdgeColor', Color_touch_win, 'LineWidth', 1);  \n    \n    elseif strcmp(Name1, 'white')\n        plot(Xw(touch), 480 - Yw(touch), 'o', 'MarkerSize', 15, 'MarkerEdgeColor', Color_touch_win, 'LineWidth', 1);\n    \n    end\n\nelse                                  % soit on gagne soit ou perd.         Mais elseif inside because we can have Name1 = 'No ball moved'.\n    \n    if strcmp(Name1, 'red')\n        plot(Xr(touch), 480 - Yr(touch), 'o', 'MarkerSize', 15, 'MarkerEdgeColor', Color_touch_loose, 'LineWidth', 1);\n    \n    elseif strcmp(Name1, 'yellow')\n        plot(Xy(touch), 480 - Yy(touch), 'o', 'MarkerSize', 15, 'MarkerEdgeColor', Color_touch_loose, 'LineWidth', 1);  \n    \n    elseif strcmp(Name1, 'white')\n        plot(Xw(touch), 480 - Yw(touch), 'o', 'MarkerSize', 15, 'MarkerEdgeColor', Color_touch_loose, 'LineWidth', 1);\n    \n    end\nend\n\n% Mise en forme du graphique\naxis equal; % Assure un ratio 1:1\naxis off;   % Cache les axes x/y\nset(gca, 'Color', 'w'); % Fond blanc\nset(gcf, 'Color', 'w');\nset(gcf, 'InvertHardcopy', 'off'); % Garde le fond blanc lors de la sauvegarde, pour empecher de mauvaise surprise\n\n% Le titre\ntitleStr = sprintf('Scores sheet - %s - (%s)', filename, SeqDateTime);\ntitle(titleStr, 'Color', 'k', 'FontSize', 14, 'FontWeight', 'bold');\n\n% Ajouter les annotations de texte (en bas)\nY_txt_line1 = Ymax + 10;\nY_txt_line2 = Ymax + 50;\nY_coord1 = 480 - Y_txt_line1;\nY_coord2 = 480 - Y_txt_line2;       %480 - : pour rammener le Y à notre repère classique\n\n\n\n\n\nwinnerStr = sprintf('Score sheet for \"%s\"\\n %s', Name1, WinLose);\ntext(Xmin, Y_coord1, winnerStr, 'Color', 'k', 'FontSize', 10, 'VerticalAlignment', 'top');\n\ndistStrR = sprintf('red_d:%dpx', round(PathR));\ntext(Xmin, Y_coord2, distStrR, 'Color', 'k', 'FontSize', 10, 'VerticalAlignment', 'top');             \n\ndistStrY = sprintf('yellow_d:%dpx', round(PathY));\ntext(Xmax / 2, Y_coord2, distStrY, 'Color', 'k', 'FontSize', 10, 'VerticalAlignment', 'top');\n\ndistStrW = sprintf('white_d:%dpx', round(PathW));\ntext(Xmax, Y_coord2, distStrW, 'Color', 'k', 'FontSize', 10, 'VerticalAlignment', 'top', 'HorizontalAlignment', 'right');\n\nsummaryStr = sprintf('%d ball(s) moved\\n%d band(s) touched', NbBallsMoved, touch_nb);\ntext(Xmax, Y_coord1, summaryStr, 'Color', 'k', 'FontSize', 10, 'VerticalAlignment', 'top', 'HorizontalAlignment', 'right');\n\nhold off;\n\n% 5. SAUVEGARDE DES RÉSULTATS\n\n\n% Sauvegarder l'image en PDF\nPdfFileName = sprintf('ScoreSheet%s.pdf', filename);    \nprint(fig, PdfFileName, '-dpdf', '-fillpage');\nfprintf('Graphique sauvegardé sous le nom : %s\\n', PdfFileName);\n\n% Sauvegarder le résumé en TXT\ntxtFileName = sprintf('Summary%s.txt', filename);\nfid = fopen(txtFileName, 'w');\nif fid == -1\n    error('Impossible de créer le fichier TXT.');\nend\n\n\n\nfprintf(fid, 'f:%s; ',Name1txt);\nfprintf(fid, 's:%s; ',WinLosetxt);\nfprintf(fid, 'n:%d; ',NbBallsMoved);\nfprintf(fid, 'b:%d; ',touch_nb);\nfprintf(fid, 'rb:%d; ',round(PathR));\nfprintf(fid, 'yb:%d; ',round(PathY));\nfprintf(fid, 'wb:%d; ',round(PathW));\n\n\n\nfclose(fid);\nfprintf('Résumé sauvegardé sous le nom : %s\\n', txtFileName);\n\n\n\n% ########################################################################\n%\n%  DEFINITION DES FONCTIONS LOCALES\n%\n% ########################################################################\n\n\n% EXO 4\nfunction [X, Y] = InterpolateNan(X,Y)\n    added_start = false;\n    added_end = false;    % on ajoute au début ou à la fin un zéro pour éviter les problèmes de bords.\n    if isnan(X(1))\n        X = [0 , X];\n        Y = [0 , Y];\n        added_start = true;\n    end\n    \n    if isnan(X(end))\n        X(end + 1) = 0;\n        Y(end + 1) = 0;\n        added_end = true; \n    end\n    \n    idx_connus_X = find(~isnan(X));\n    \n    valeurs_connues_X = X(idx_connus_X);\n    \n    idx_tous_X = 1:length(X);\n    X = interp1(idx_connus_X, valeurs_connues_X, idx_tous_X, 'next');\n    \n    idx_connus_Y = find(~isnan(Y));\n    \n    valeurs_connues_Y = Y(idx_connus_Y);\n    \n    idx_tous_Y = 1:length(Y);\n    Y = interp1(idx_connus_Y, valeurs_connues_Y, idx_tous_Y, 'next');\n    \n    if added_start\n        X = X(2:end);\n        Y = Y(2:end);\n    end\n    if added_end\n        X = X(1:end-1);\n        Y = Y(1:end-1);\n    end\n    \nend\n\n\n% Note : On considère que le premier élément ne peut pas être un outlier.\n\nfunction[X,Y] = RemoveOutlier(X, Y)\n\noutlierX = isoutlier(X, 'movmedian', 10);\noutlierY = isoutlier(Y, 'movmedian', 10);\n\noutlierX([1 end]) = false;\noutlierY([1 end]) = false; \n\nidx_out_X = find(outlierX);        % done les index ou ya les outliers dans X\nX(idx_out_X) = X(idx_out_X - 1);   % remplace valeur outlier par precedente valeur ie (-1)\n\nidx_out_Y = find(outlierY);         % pas de risque de index out of range  car (1) et (end) = false dans le logical array\nY(idx_out_Y) = Y(idx_out_Y - 1);    % pas de problème de faire juste -1 car il n'y a pas de groupe d'outliers.\n\n\nend\n\n\n\n% EXO 2\nfunction [Xmin, Xmax, Ymin, Ymax] = GetFrame(Xr, Yr, Xy, Yy, Xw, Yw)\n    all_X = [Xr, Xy, Xw];\n    all_Y = [Yr, Yy, Yw];\n    \n    Xmin = min(all_X);\n    Xmax = max(all_X);    %calcul min et max global\n    Ymin = min(all_Y);\n    Ymax = max(all_Y);\nend\n\n\nfunction PathLength = GetBallPathLength(X,Y)\n    \n    norme = sqrt(diff(X).^2 + diff(Y).^2);\n    PathLength = sum(norme); \n\nend\n\n\n\nfunction [FirstMoveIdx, MoveDist] = GetFirstMoveIdx(X, Y, MoveDistPx)\n   \n\n    MoveDist = sqrt(diff(X.^2) + diff(Y.^2));    % les segments(distances) entre chaque positions consécutives, pour utiliser après pour trouver FirstBall\n                                                 \n                                                 \n                                                 \n    X = X - X(1);                        % changement de référentiel                                             \n    Y = Y - Y(1);\n    distance = sqrt(X.^2 + Y.^2);        % ici pas besoin de faire diff() car distance par rapport à X(1) et Y(1), pas entre positions consécutives \n                                                                           \n    FirstMoveIdx = find(distance > MoveDistPx, 1 , 'first');   % prend le premier indice tel que la distance > MoveDistPix \n    \n\nend\n\n\n\n% EXO 3\nfunction [IdxTouch] = GetTouchIdx(X, Y, Xmin, Xmax, Ymin, Ymax, BallBorderDist)\n\n    idxLeft = find(X - Xmin <= BallBorderDist);\n    idxRight = find(Xmax - X <= BallBorderDist);     \n    idxTop = find(Y - Ymin <= BallBorderDist);       \n    idxBottom = find(Ymax - Y <= BallBorderDist); \n\n    % Dans cette fonction, il y a 2 choses à checker. Si deux bords sont hit\n    % successivement et si deux boules satisfont la condition du find.\n    % Ce sont deux cas différents, qu'on ne peut pas checker d'un seul coup.\n    % On commence d'abord par checker chaque bord seul si on a des index\n    % successifs. Sinon, si je check après tout avoir mis ensemble, je risque\n    % de perdre des rebonds sur des bords successifs, qui se feront passer\n    % pour des doublons qui satisfont la condition <= BallBorder Dist\n   \n                                                                                                           \n    if ~isempty(idxLeft)                                   \n        idxLeft = idxLeft([true, diff(idxLeft) > 1]);      % true, c'est pour ajouter true au vecteur logique au début, comme ça on ne prend que le 1er indice détecté\n    end\n    if ~isempty(idxRight) \n        idxRight = idxRight([true, diff(idxRight) > 1]);                                                 \n    end\n    if ~isempty(idxTop) \n        idxTop = idxTop([true, diff(idxTop) > 1]);            \n    end\n    if ~isempty(idxBottom) \n        idxBottom = idxBottom([true, diff(idxBottom) > 1]);    \n    end\n               \n    [IdxTouch] = [idxLeft idxRight idxTop idxBottom];  % on fusionne le tout\n    [IdxTouch] = unique(IdxTouch);  % enlève les doublons éventuels et trie en ordre croissant.            \n   \n    IdxTouch(IdxTouch == 1) = [];             % On enlève index = 1, car une balle peut déjà être sur le bord au début de la partie.\n  \nend\n\n\n                                                     \nfunction [FirstBall,SecondBall,LastBall, NbBallsMoved] = GetBallMoveOrder(Xr, Yr, Xy, Yy, Xw, Yw, MoveDistPx)\n\n    def_idx = [1 2 3];     % red = 1, yellow = 2 , white = 3\n    \n    [idxR,segsR] = GetFirstMoveIdx(Xr, Yr, MoveDistPx);\n    [idxY,segsY] = GetFirstMoveIdx(Xy, Yy, MoveDistPx);        \n    [idxW,segsW] = GetFirstMoveIdx(Xw, Yw, MoveDistPx);\n    \n    len = length(Xr);                       % Longueur de référence\n    if isempty(idxR), idxR = len + 1; end\n    if isempty(idxY), idxY = len + 1; end   % On donne valeur impossible, et on ne garde pas vide puisque sinon, on ne pourra pas trier par la suite.\n    if isempty(idxW), idxW = len + 1; end\n    \n    d1R = 0;\n    d1Y = 0;  % variable pour stocker distance initial parcourue\n    d1W = 0;\n\n    % fprintf('idxR=%s, idxY=%s, idxW=%s\\n', mat2str(idxR), mat2str(idxY), mat2str(idxW)); \n    \n    if ~isempty(segsR), d1R = segsR(1); end      % On garde juste 1er segment / distance initiale parcourue, d'où (1)\n    if ~isempty(segsY), d1Y = segsY(1); end      % Si non vide, donne aux variables distance initale parcourue, sinon reste 0\n    if ~isempty(segsW), d1W = segsW(1); end\n    \n    % fprintf('d1R=%.3f, d1Y=%.3f, d1W=%.3f\\n', d1R, d1Y, d1W);\n\n    store_idx = [idxR idxY idxW];                                                                           \n    store_d1 = [d1R d1Y d1W];                 \n                                                 % sortrows() : On utilise le tri des élements des colonnes pour bouger les lignes de la matrice                                                                  \n    M = [store_idx(:) store_d1(:) def_idx(:)];   % Tri d'abord selon la colonne 1 dans l'ordre croissant, boule qui bouge en premier a le plus petit indice et donc est au début de la colonne 1     \n    M = sortrows(M, [1 -2]);                     % Ensuite, si deux lignes on la même valeur dans la colonne 1 i.e: on a le meme indice, alors on trie encore la matrice suivant la 2eme colonne\n                                                 % Et dans ce cas, les seules lignes qui bougent sont celles où dans la colonne 1 y'a eu une égalité\n                                                 \n                                                 % Le - c'est juste pour\n                                                 % trier dans l'ordre\n                                                 % décroissant les\n                                                 % distances initiales, car\n                                                 % on veut la plus grande\n                                                 % distance initiale\n                                                 % parcourue.\n\n\n\n    moved_idx = M(M(:,1) <= len, 3).'; % Filtre en utilisant len (et donc len + 1 impossible d'être pris) pour enfin trouver l'ordre des boules\n    NbBallsMoved = numel(moved_idx);\n\n\n    %disp(moved_idx);\n    %disp(d1R);                        \n    %disp(d1Y);           % to test intermediate values\n    %disp(d1W);\n\n    FirstBall = 0; SecondBall = 0; LastBall = 0;\n    \n    if NbBallsMoved >= 1, FirstBall = moved_idx(1); end     \n    if NbBallsMoved >= 2, SecondBall = moved_idx(2); end\n    if NbBallsMoved >= 3, LastBall = moved_idx(3); end\n   \nend\n\n\n\n% Version 26 Decembre 10:30 PM " ("string")) -> (w47:string)
  "script matlab" <- w47
  n24 = Current VI's Path() -> (path=w60:path)
  n25 = Strip Path(path=w60) -> (stripped path=w59:path)  [unwired: 1 out]
  n26 = Format Into String(format string="Analyse%s.m", "filename") -> (resulting string=w56:string)  [unwired: 2 in, 1 out]
  n27 = Build Path(base path=w59, name or relative path=w56) -> (appended path=w48:path)
  "matlab path" <- w48
  n28 = Open/Create/Replace File(file path (use dialog)=w48, error in="error in", operation (0:open)=T1."replace or create") -> (refnum out=w54:refnum<file>, error out=w52:errorcluster)  [unwired: 3 in, 1 out]
  n29 = Write to Text File(file (use dialog)=w54, text=w47, error in=w52) -> (refnum out=w53:refnum<file>, error out=w51:errorcluster)  [unwired: 1 in, 1 out]
  n30 = Close File(refnum=w53, error in=w51) -> (error out=→"error out":errorcluster)  [unwired: 1 out]
